vi "Step Types Mind Map.vi"() -> ()   [LabVIEW 2020, in "MacroAssert.lvlib"]
uses:
  MacroAssert.lvlib
panel:
  in  "Mouse Action":T1(ring)
  in  "Tree":string(tree)
  # "Mouse action params:\n\nButton: left/right/middle\nClick type: normal/hold/release\nModifiers: Ctrl/Alt/Shift\nAbsolute/relative coords\nClick control? Ctl name\n\nFor move or move & click:\nscreen/window/ctl?"
  # "Keyboard action params:\n\nKey delay\nModifiers: Ctrl/Alt/Shift"
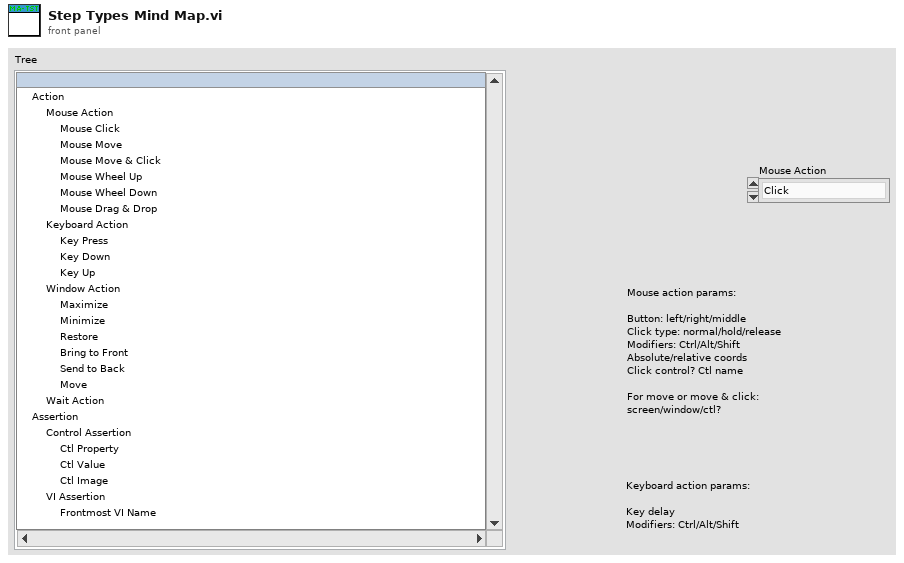
[diagram p1: front panel]
types:
  T1 = enum16{"Click", "Move", "Move and Click", "Wheel Up", "Wheel Down", "Drag and Drop"}
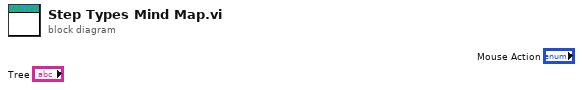
[diagram p0: block diagram]
diagram:
